vi "Bind Multiple Terminal Values.vi"(4 "Ignore Past Updates? (F)":bool, 6 "Value Changes Only? (T)":bool=TRUE, 8 "error in (no error)":errorcluster, 10 "Ctl Refnums":refnum<vi>[](array[refnum]), 11 "IViewable in":refnum<class "IViewable.lvclass">) -> (0 "error out":errorcluster, 3 "IViewable out":refnum<class "IViewable.lvclass">)   [LabVIEW 2017, in "IViewable.lvlib" / "IViewable.lvclass"]
doc: "Bind multiple control terminal values (controls or indicators) to published data whose name and type match those of the wired terminal references."
uses:
  IViewable.lvclass
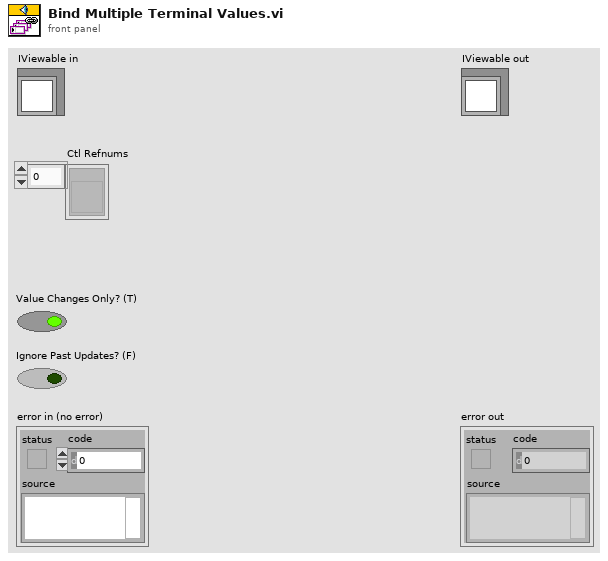
[diagram p1: front panel]
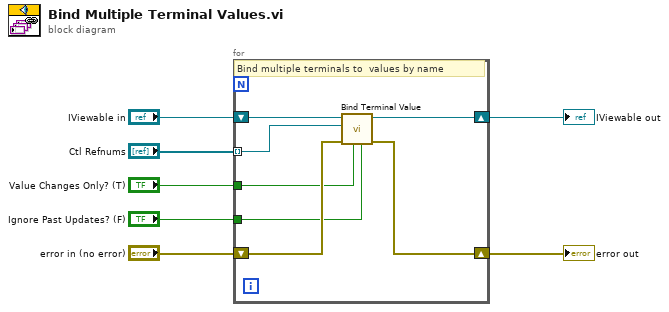
[diagram p0: block diagram]
diagram:
  n1 = for {
    shift-right: [w13] -> w6
    shift-left: "IViewable in" -> [w14]
    shift-right: [w11] -> w4
    shift-left: "error in (no error)" -> [w12]
    tunnel: "Ctl Refnums" -> [w10] mode=indexing
    tunnel: "Value Changes Only? (T)" -> [w9]
    tunnel: "Ignore Past Updates? (F)" -> [w8]
    # "Bind multiple terminals to  values by name"
    n2 = call "Bind Terminal Value.vi"("Ignore Past Updates? (F)"=w8, "Value Changes Only? (T)"=w9, "error in (no error)"=w12, "Ctl Refnum"=w10, "IViewable in"=w14) -> ("error out"=w11:errorcluster, "IViewable out"=w13:refnum<class "IViewable.lvclass">)  [unwired: 5 in]
  }
  "error out" <- w4
  "IViewable out" <- w6
